vi "Configure Modulation Waveform Advanced.vi"   [LabVIEW 2014, in "Agilent PSG MXG Series.lvlib"]
doc: "Configures parameters for dual-sine or swept-sine waveform for N5171B, N5172B, N5181B, N5182B."
uses:
  Agilent PSG MXG Series.lvlib
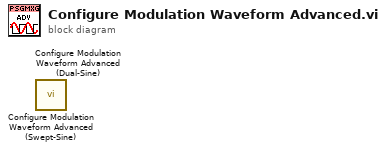
[diagram p0: block diagram]
diagram:
  n1 = call "Configure Modulation Waveform Advanced (Swept-Sine).vi"() -> ()  [unwired: 14 in, 2 out]
  n2 = call "Configure Modulation Waveform Advanced (Dual-Sine).vi"() -> ()  [unwired: 14 in, 2 out]
